vi "Set Two Movables.vi"(9 "Movable 2 in":refnum<class "Game Board Component.lvclass">, 10 "Movable 1 in":refnum<class "Game Board Component.lvclass">, 11 "Collision in":refnum<class "Collision.lvclass">) -> (3 "Collision out":refnum<class "Collision.lvclass">)   [LabVIEW 2021, in "Collision.lvclass"]
doc: "MIT Licence\nCopyright (c) 2024 David Grollier"
uses:
  Collision.lvclass
  Game Componants/Game Board Component/Game Board Component.lvclass
  Collision.lvclass/Collision.ctl
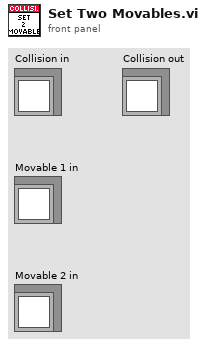
[diagram p1: front panel]
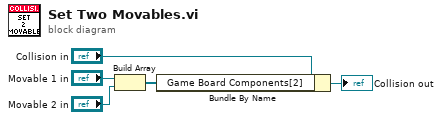
[diagram p0: block diagram]
diagram:
  n1 = Build Array("Movable 1 in", "Movable 2 in") -> (w2:refnum<class "Game Board Component.lvclass">[])
  n2 = Bundle By Name(cluster="Collision in", "Game Board Components[2]"=w2) -> (→"Collision out":refnum<class "Collision.lvclass">)
